vi "Brown--constant.vi"() -> ()   [LabVIEW 2018]
panel:
  out "Color":u32(colorbox)
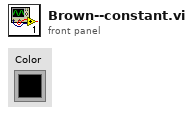
[diagram p1: front panel]
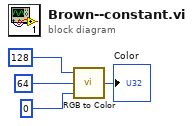
[diagram p0: block diagram]
diagram:
  n1 = call <vilib>:"RGB to Color.vi"("B"=u8 0, "G"=u8 64, "R"=u8 128) -> ("Color"=→"Color":u32)
